vi "Advance past next JSON Value (inlined COPY).vi"(7 "JSON":string, 9 "Offset":i32, 11 "State":T2=enum."Leading Whitespace") -> (0 "JSON Value Type":T1, 1 "Offset":i32, 3 "State":T2=enum."Value end", 4 "Type":T2, 6 "Value start":i32)   [LabVIEW 2017, in "JSONtext.lvlib"]
uses:
  JSONtext.lvlib
  Parsing State.ctl
  JSON Value Type.ctl
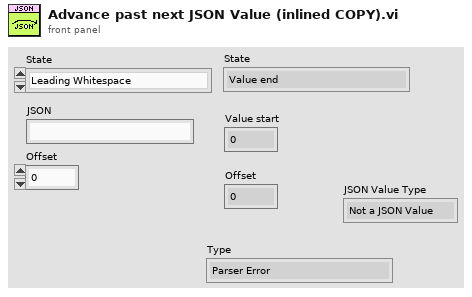
[diagram p1: front panel]
types:
  T1 = typedef "JSONtext.lvlib/JSON Value Type.ctl" = enum16{"Not a JSON Value", "JSON Object", "JSON Array", "String", "Number", "true", "false", "null"}
  T2 = typedef "JSONtext.lvlib/Parsing State.ctl" = enum16{"Parser Error", "Object", "Array", "String", "Number/Other", "Leading Whitespace", "Object end", "Array end", "Value end"}
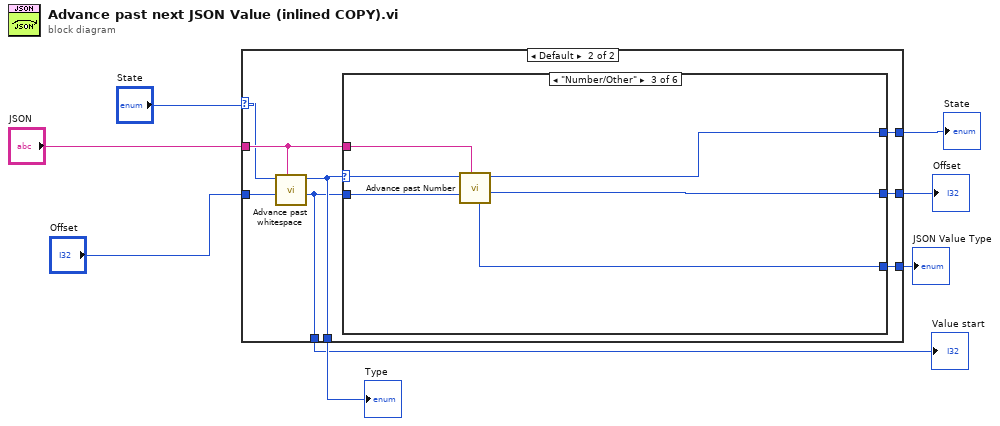
[diagram p0: block diagram]
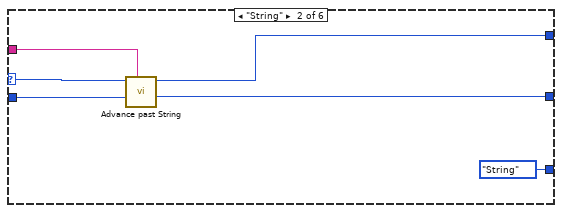
[diagram p4: hidden frame]
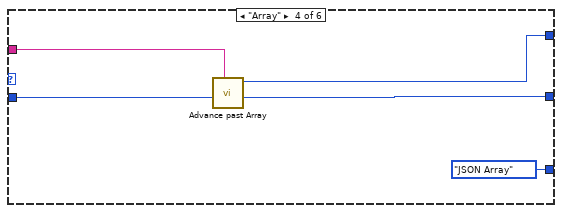
[diagram p5: hidden frame]
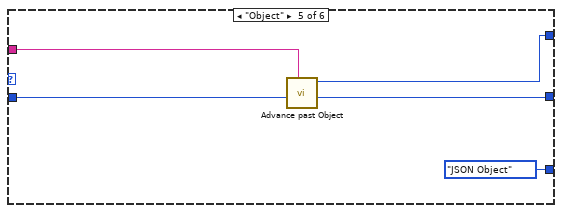
[diagram p6: hidden frame]
diagram:
  n1 = case shown="Default" "State" {
    selector: "State" -> [w9 w12]
    tunnel: "JSON" -> [_ w18]
    tunnel: [w9 w17] -> w7
    tunnel: [w10 w16] -> w6
    tunnel: [w9 w15] -> w5
    tunnel: "Offset" -> [w10 w14]
    tunnel: [w10 w13] -> w3
    tunnel: [_ w11] -> w1
    frame "Parser Error" {
    }
    frame Default {
      n2 = call "Advance past whitespace.vi"("JSON"=w18, "Offset"=w14, "Parser State in"=w12) -> ("Offset of first non-whitespace"=w13:i32, "Parser State"=w17:T2)  [unwired: 7 in]
      n3 = case shown="\"Number/Other\"" w17 {
        selector: w17 -> [w19 w25 w31 _ _ w43]
        tunnel: w18 -> [_ w26 w32 w34 w39 _]
        tunnel: w13 -> [w20 w24 w30 w35 w42 w44]
        tunnel: [w20 w23 w29 w36 w40 w44] -> w16
        tunnel: [w19 w22 w28 w37 w41 w43] -> w15
        tunnel: [_ JSON_Value_Type."String" ("JSON Value Type") w27 JSON_Value_Type."JSON Array" ("JSON Value Type") JSON_Value_Type."JSON Object" ("JSON Value Type") _] -> w11
        frame "Parser Error", Default {
        }
        frame "String" {
          n4 = call "Advance past String.vi"("JSON"=w26, "Offset"=w24, "State in"=w25) -> ("Offset past match"=w23:i32, "State"=w22:T2)  [unwired: 6 in, 1 out]
        }
        frame "Number/Other" {
          n5 = call "Advance past Number.vi"("JSON"=w32, "Offset (0)"=w30, "Parser State in"=w31) -> ("Offset past match"=w29:i32, "Parser State"=w28:T2, "JSON Value Type"=w27:T1)  [unwired: 5 in, 1 out]
        }
        frame "Array" {
          n6 = call "Advance past Array.vi"("JSON"=w34, "Offset"=w35) -> ("Offset past Array"=w36:i32, "State"=w37:T2)  [unwired: 7 in, 1 out]
        }
        frame "Object" {
          n7 = call "Advance past Object.vi"("JSON"=w39, "Offset"=w42) -> ("Offset past Object"=w40:i32, "State"=w41:T2)  [unwired: 7 in, 1 out]
        }
        frame "Value end" {
        }
      }
    }
  }
  "State" <- w5
  "Offset" <- w6
  "Value start" <- w3
  "Type" <- w7
  "JSON Value Type" <- w1
